vi "Get Stream.vi"(8 "error in (no error)":errorcluster, 11 "Endpoint in":refnum<class "Endpoint.lvclass">) -> (0 "error out":errorcluster, 2 "Stream":refnum<class "Stream.lvclass">, 3 "Endpoint out":refnum<class "Endpoint.lvclass">)   [LabVIEW 2020, in "Stream-Simple-Msg.lvlib" / "Endpoint.lvclass"]
uses:
  Endpoint.lvclass
  <vilib>/IlluminatedG/lv-stream/stream/Stream.lvclass
  Endpoint.lvclass/Endpoint.ctl
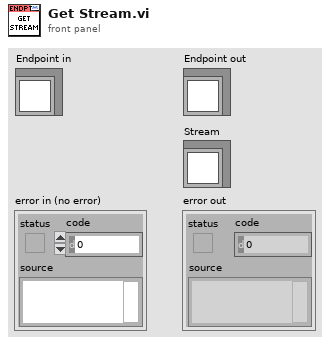
[diagram p1: front panel]
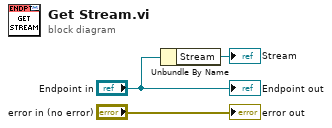
[diagram p0: block diagram]
diagram:
  n1 = Unbundle By Name("Endpoint in") -> ("Stream"=→"Stream":refnum<class "Stream.lvclass">)
  "error out" <- "error in (no error)"
  "Endpoint out" <- "Endpoint in"
